vi "for loop.vi"() -> ()   [LabVIEW 2014]
panel:
  out "indicator":i32
  in  "input":dbl format="%#_13g"
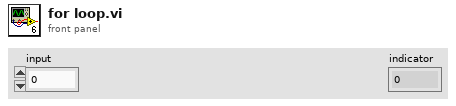
[diagram p1: front panel]
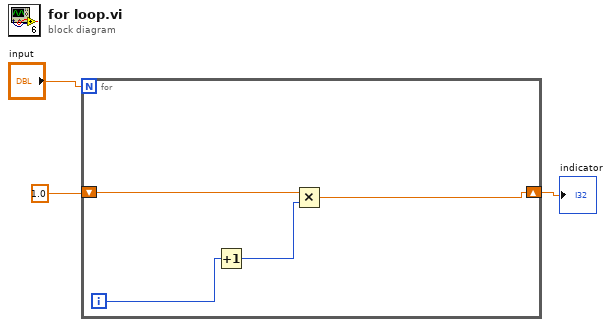
[diagram p0: block diagram]
diagram:
  n1 = for {
    N: "input" -> [_]
    shift-right: [w6] -> w1
    shift-left: 1.0 -> [w7]
    i -> [w5]
    n2 = Increment(x=w5) -> (x+1=w4:i32)
    n3 = Multiply(x=w7, y=w4) -> (x*y=w6:dbl)
  }
  "indicator" <- w1
